vi "Reset_Instr.vi"(8 "error in (no error)":errorcluster caption="entrée d'erreur (pas d'erreur)", 11 "Class Instrument Multimeter en entrée":refnum<class "Class Instrument Balance.lvclass">) -> (0 "error out":errorcluster caption="sortie d'erreur", 3 "Class Instrument Multimeter en sortie":refnum<class "Class Instrument Balance.lvclass">)   [LabVIEW 2020, in "Library Instrument & Equipement.lvlib" / "Library Instruments.lvlib" / "Class Instrument Balance.lvclass"]
uses:
  Class Instrument Balance.lvclass
  Class Instrument Balance.lvclass/Class Instrument Balance.ctl
  Instrument (Default)/Class Instrument (Default).lvclass
  Balance/Balance (Default)/Class Balance (Default).lvclass
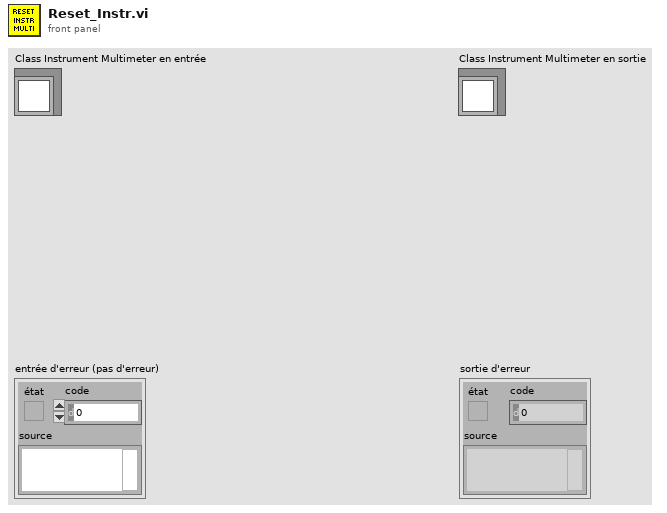
[diagram p1: front panel]
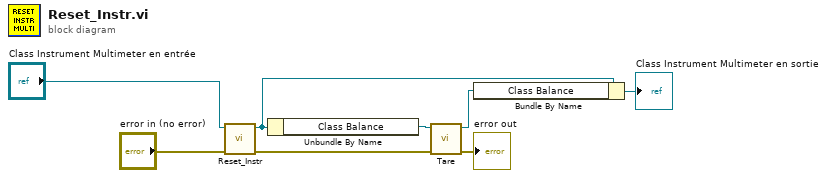
[diagram p0: block diagram]
diagram:
  n1 = call-parent "Reset_Instr.vi"("error in (no error)"="error in (no error)", "Class Instrument (Default) en entrée"="Class Instrument Multimeter en entrée") -> ("error out"=w4:errorcluster, "Class Instrument (Default) en sortie"=w6:refnum<class "Class Instrument Balance.lvclass">)  [unwired: 8 in]
  n2 = Unbundle By Name(w6) -> ("Class Balance"=w1:refnum<class "Class Balance (Default).lvclass">)
  n3 = call-dynamic "Tare.vi"("error in (no error)"=w4, "Class Balance (Default) en entrée"=w1) -> ("error out"=→"error out":errorcluster, "Class Balance (Default) en sortie"=w2:refnum<class "Class Balance (Default).lvclass">)  [unwired: 8 in]
  n4 = Bundle By Name(cluster=w6, "Class Balance"=w2) -> (→"Class Instrument Multimeter en sortie":refnum<class "Class Instrument Balance.lvclass">)
